vi "Config AO.vi"(6 "Channel config":T1, 7 "Output range":cluster{"output high":dbl, "output low":dbl}={"output high"=1.5, "output low"=0.0}, 8 "error in":errorcluster, 11 "task in":refnum<k21>) -> (0 "error out":errorcluster, 3 "task out":refnum<k21>)   [LabVIEW 2019]
doc: "This example demonstrates how to acquire a continuous amount of data (Waveform) using the DAQ device's internal clock. It also shows how to synchronize two devices for different device families (E Series, S Series, M Series, X Series, DSA, and SC Express), to simultaneously acquire the data.\n\nFor instructions on how to connect your signals to the DAQ device, refer to your device documentation."
uses:
  <vilib>/DAQmx/create/channels.llb/DAQmx Create Channel (AO-Voltage-Basic).vi
panel:
  # "Config AO"
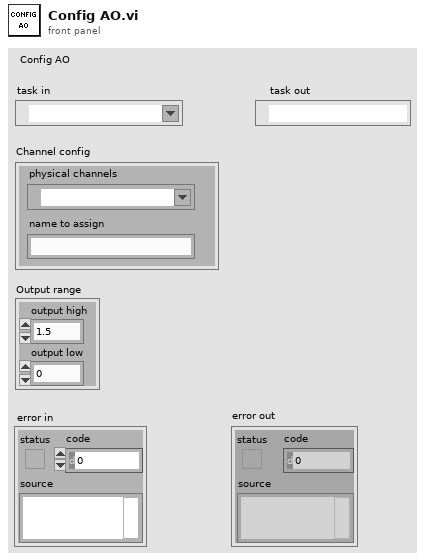
[diagram p1: front panel]
types:
  T1 = cluster{"physical channels":tag, "name to assign":string}
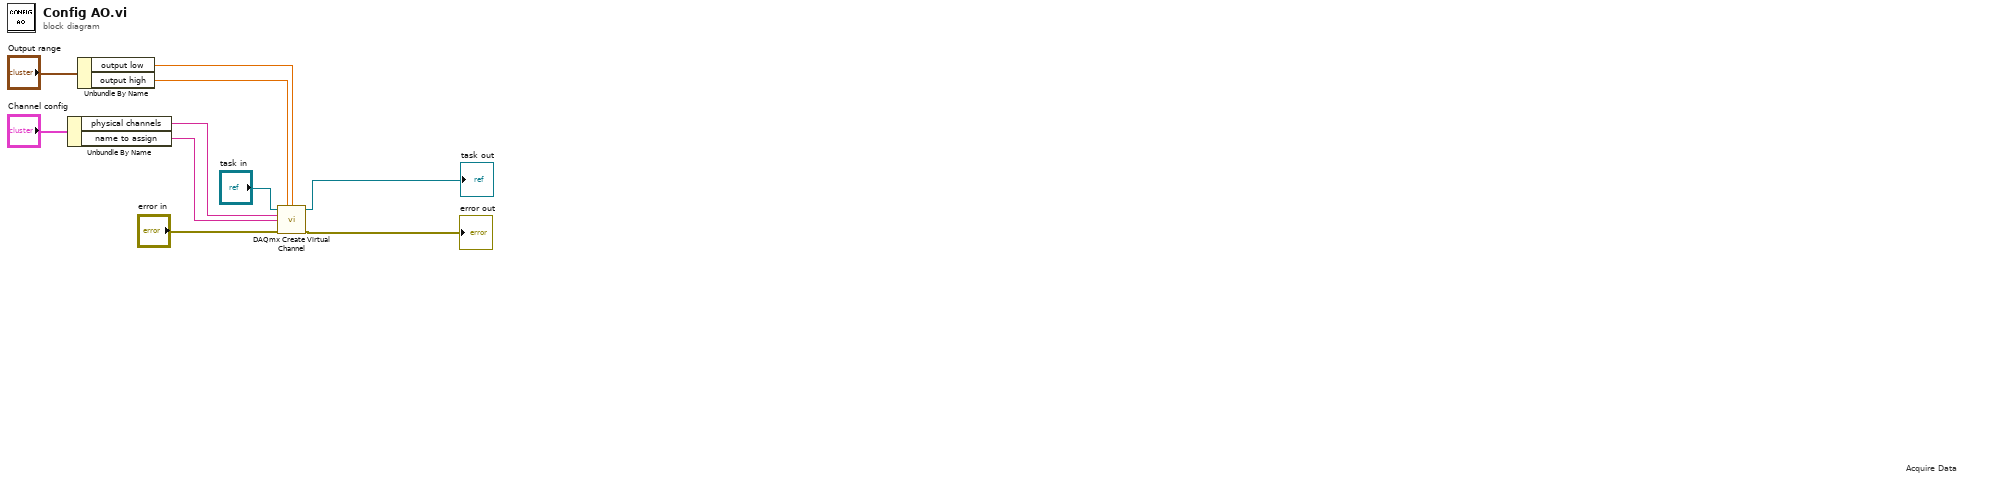
[diagram p0: block diagram]
diagram:
  # "Acquire Data"
  n1 = Unbundle By Name("Channel config") -> ("physical channels"=w7:tag, "name to assign"=w6:string)
  n2 = Unbundle By Name("Output range") -> ("output low"=w2:dbl, "output high"=w1:dbl)
  n3 = call-poly <vilib>:"DAQmx Create Virtual Channel.vi"("task in"="task in", "maximum value"=w1, "minimum value"=w2, "physical channels"=w7, "name to assign"=w6, "error in"="error in") -> ("task out"=→"task out":refnum<k21>, "error out"=→"error out":errorcluster)  [unwired: 8 in]
